vi "VNA_Set_Trace_Def.vi"(2 "error in (no error)":errorcluster, 3 "Index":u8, 4 "Def":T1(ring), 5 "VISA resource name":refnum<visa-resource-name>) -> (0 "error out":errorcluster, 1 "VISA VNA out":refnum<visa-resource-name>)   [LabVIEW 2017]
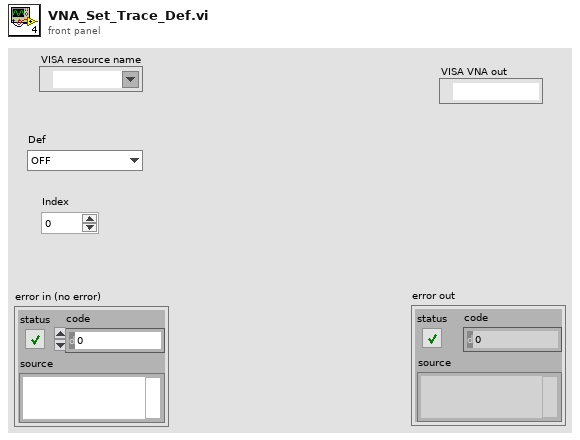
[diagram p1: front panel]
types:
  T1 = enum16{"OFF", "S11", "S21", "S12", "S22", "A", "B", "C", "D", "R1", "R2", "AUX1", "AUX2"}
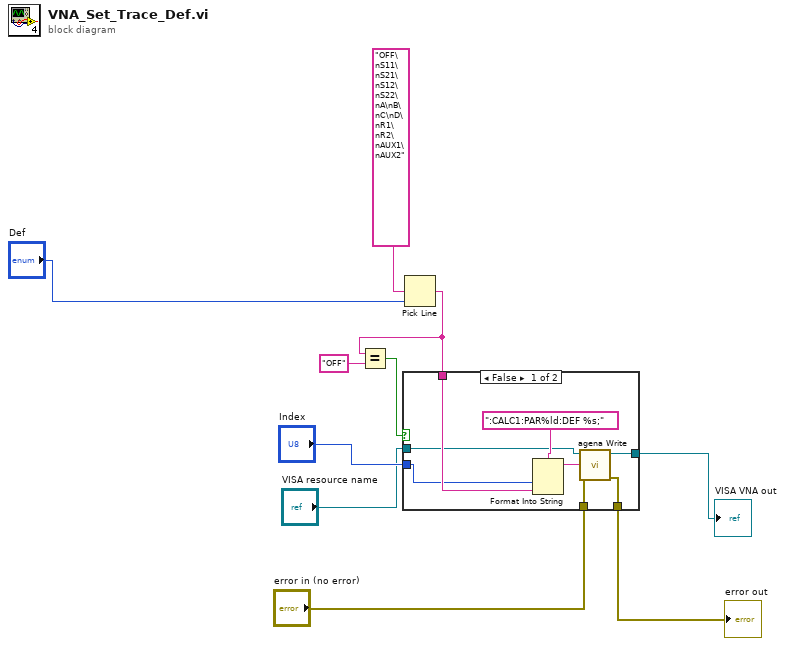
[diagram p0: block diagram]
diagram:
  n1 = Pick Line(multi-line string="OFF\nS11\nS21\nS12\nS22\nA\nB\nC\nD\nR1\nR2\nAUX1\nAUX2", line index="Def") -> (output string=w8:string)  [unwired: 1 in]
  n2 = Equal?(x=w8, y="OFF") -> (x = y?=w6:bool)
  n3 = case shown="False" w6 {
    tunnel: w8 -> [w17 _]
    tunnel: "Index" -> [w16 _]
    tunnel: "error in (no error)" -> [w15 w19]
    tunnel: "VISA resource name" -> [w13 w20]
    tunnel: [w12 w19] -> w3
    tunnel: [w11 w20] -> w2
    frame False {
      n4 = Format Into String(format string=":CALC1:PAR%ld:DEF %s;", w16, w17) -> (resulting string=w14:string)  [unwired: 2 in, 1 out]
      n5 = call "agena Write.vi"("error in (no error)"=w15, "String ()"=w14, "VISA resource name"=w13) -> ("error out"=w12:errorcluster, "VISA resource name out"=w11:refnum<visa-resource-name>)  [unwired: 6 in, 1 out]
    }
    frame True {
    }
  }
  "VISA VNA out" <- w2
  "error out" <- w3
